vi "EEG_2022_040_LabView_3.6.vi"(8 "Error In":errorcluster, 9 "Min.  Temperature":dbl, 10 "Max.  Temperature":dbl, 11 "Current  Temperatue":dbl) -> (0 "Error out":errorcluster, 2 "Warning Text":string, 3 "Warning?":bool)   [LabVIEW 2022 SP3]
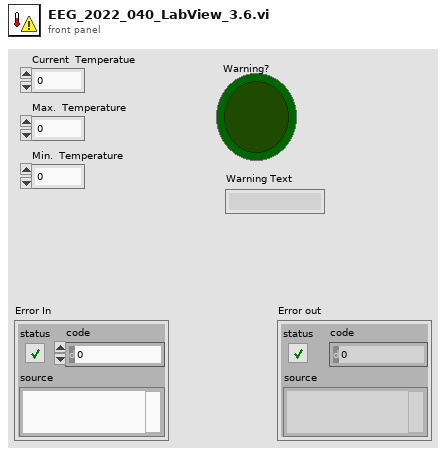
[diagram p1: front panel]
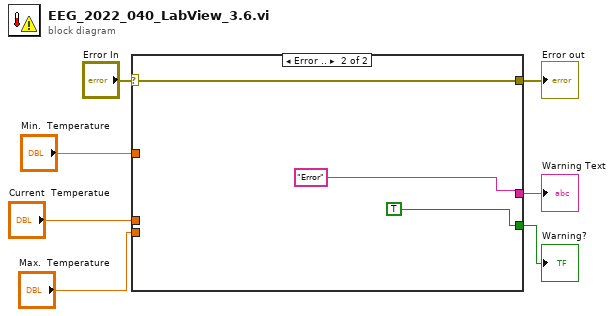
[diagram p0: block diagram]
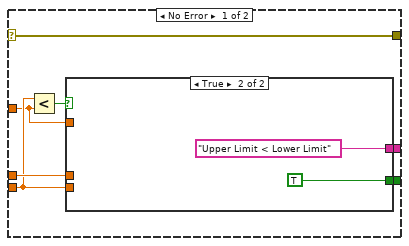
[diagram p2: hidden frame]
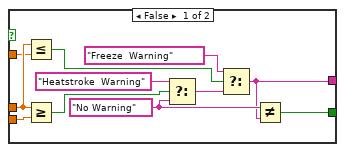
[diagram p3: hidden frame]
diagram:
  n1 = case shown="Error .." "Error In" {
    selector: "Error In" -> [w14 w28]
    tunnel: "Max.  Temperature" -> [w9 _]
    tunnel: "Current  Temperatue" -> [w13 _]
    tunnel: "Min.  Temperature" -> [w8 _]
    tunnel: [w14 w28] -> w4
    tunnel: [w11 "Error"] -> w2
    tunnel: [w10 TRUE] -> w1
    frame No Error {
      n2 = Less?(x=w9, y=w8) -> (x < y?=w12:bool)
      n3 = case shown="True" w12 {
        tunnel: w13 -> [w17 _]
        tunnel: w8 -> [w15 _]
        tunnel: w9 -> [w16 _]
        tunnel: [w19 "Upper Limit < Lower Limit"] -> w11
        tunnel: [w18 TRUE] -> w10
        frame False {
          w22 = "No Warning"
          n4 = Less Or Equal?(x=w17, y=w15) -> (x <= y?=w24:bool)
          n5 = Greater Or Equal?(x=w17, y=w16) -> (x >= y?=w23:bool)
          n6 = Select(t="Heatstroke  Warning", s=w23, f=w22) -> (s? t:f=w25:string)
          n7 = Select(t="Freeze  Warning", s=w24, f=w25) -> (s? t:f=w19:string)
          n8 = Not Equal?(x=w22, y=w19) -> (x != y?=w18:bool)
        }
        frame True {
        }
      }
    }
    frame Error {
    }
  }
  "Warning?" <- w1
  "Error out" <- w4
  "Warning Text" <- w2
